vi "Count Actors.vi"(10 "Increment?":bool) -> ()   [LabVIEW 2021, in "jettl.lvlib"]
uses:
  jettl.lvlib
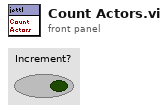
[diagram p1: front panel]
types:
  T1 = enum32{"Invalid", "Standard", "Closed", "Hidden", "Minimized", "Maximized"}
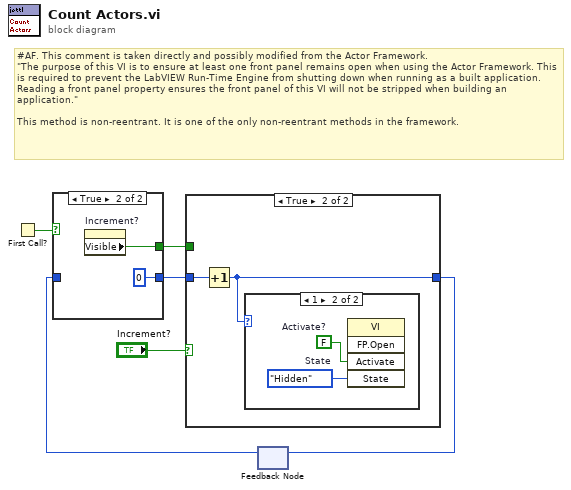
[diagram p0: block diagram]
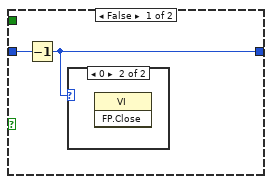
[diagram p2: hidden frame]
diagram:
  # "#AF. This comment is taken directly and possibly modified from the Actor Framework.\n\"The purpose of this VI is to ensure at least one front panel remains open when using the Actor Framework. This is required to prevent the LabVIEW Run-Time Engine from shutting down when running as a built application. Reading a front panel property ensures the front panel of this VI will not be stripped when building an application.\"\n\nThis method is non-reentrant. It is one of the only non-reentrant methods in the framework."
  n1 = First Call?() -> (First Call?: T/F=w6:bool)
  n2 = feedback #1() -> (w3:u32)  [unwired: 1 in]
  n3 = case shown="True" w6 {
    tunnel: w3 -> [w7 _]
    tunnel: [w7 u32 0] -> w5
    tunnel: [_ w8] -> w2
    frame False {
    }
    frame True {
      n4 = property on="Increment?" class="Bool (strict)"() -> ("Visible"=w8:bool)  [unwired: 2 in, 2 out]
    }
  }
  n5 = case shown="True" "Increment?" {
    tunnel: w5 -> [w11 w13]
    tunnel: [w10 w12] -> w4
    tunnel: w2 -> [_ _]
    frame False {
      n6 = Decrement(x=w11) -> (x-1=w10:u32)
      n7 = case shown="0" w10 {
        frame Default {
        }
        frame 0 {
          n8 = invoke class="VI" method="FP.Close"() -> ()  [unwired: 3 in, 3 out]
        }
      }
    }
    frame True {
      n9 = Increment(x=w13) -> (x+1=w12:u32)
      n10 = case shown="1" w12 {
        frame Default {
        }
        frame 1 {
          w14 = FALSE  # Activate?
          w15 = T1."Hidden"  # State
          n11 = invoke class="VI" method="FP.Open"("Activate"=w14, "State"=w15) -> ()  [unwired: 3 in, 5 out]
        }
      }
    }
  }
  n12 = feedback-in #1(w4) -> ()
